vi "Sets_Union(Boolean).vi"(8 "error in (no error)":errorcluster caption="错误输入（无错误）", 10 "输入数组B":bool[](array[boolean]), 11 "输入数组A":bool[](array[boolean])) -> (0 "error out":errorcluster caption="错误输出", 3 "输出数组C":bool[](array[boolean]))   [LabVIEW 2011]
uses:
  Sets_Unique(Boolean).vi
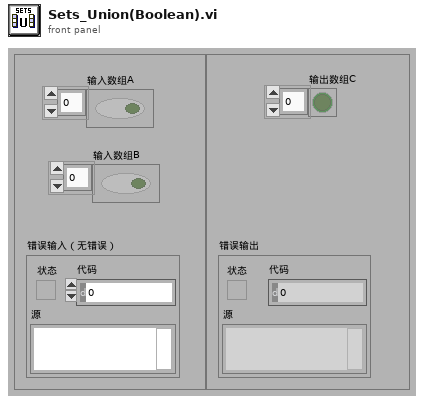
[diagram p1: front panel]
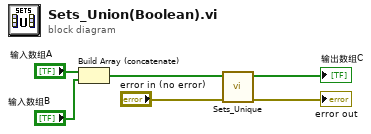
[diagram p0: block diagram]
diagram:
  n1 = Build Array (concatenate)("输入数组A", "输入数组B") -> (w3:bool[])
  n2 = call-poly "Sets_Unique.vi"("error in (no error)"="error in (no error)", "输入数组"=w3) -> ("error out"=→"error out":errorcluster, "输出数组"=→"输出数组C":bool[])  [unwired: 7 in, 1 out]
